vi "triangle.vi"() -> ()   [LabVIEW 2010]
panel:
  out "x galvo control true":u16(graph)
  out "x galvo control":u16(graph)
  in  "y resolution":u16
  out "control line counter":u16
  in  "stop":bool
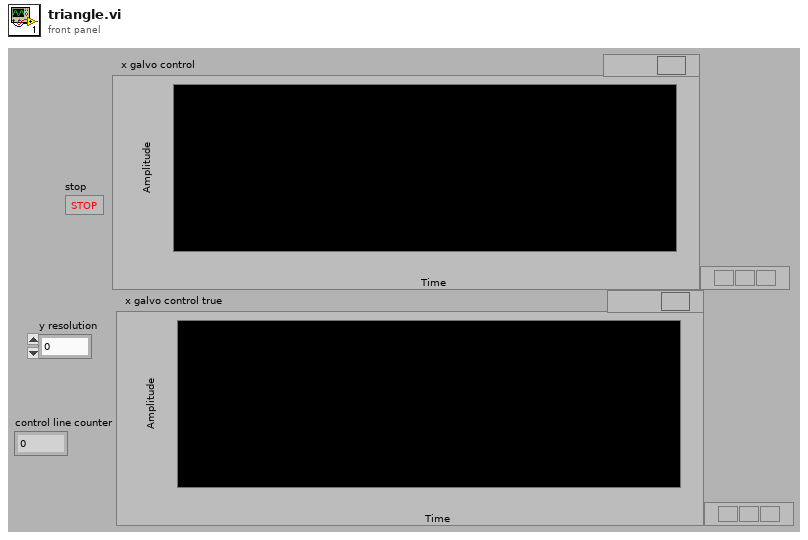
[diagram p1: front panel]
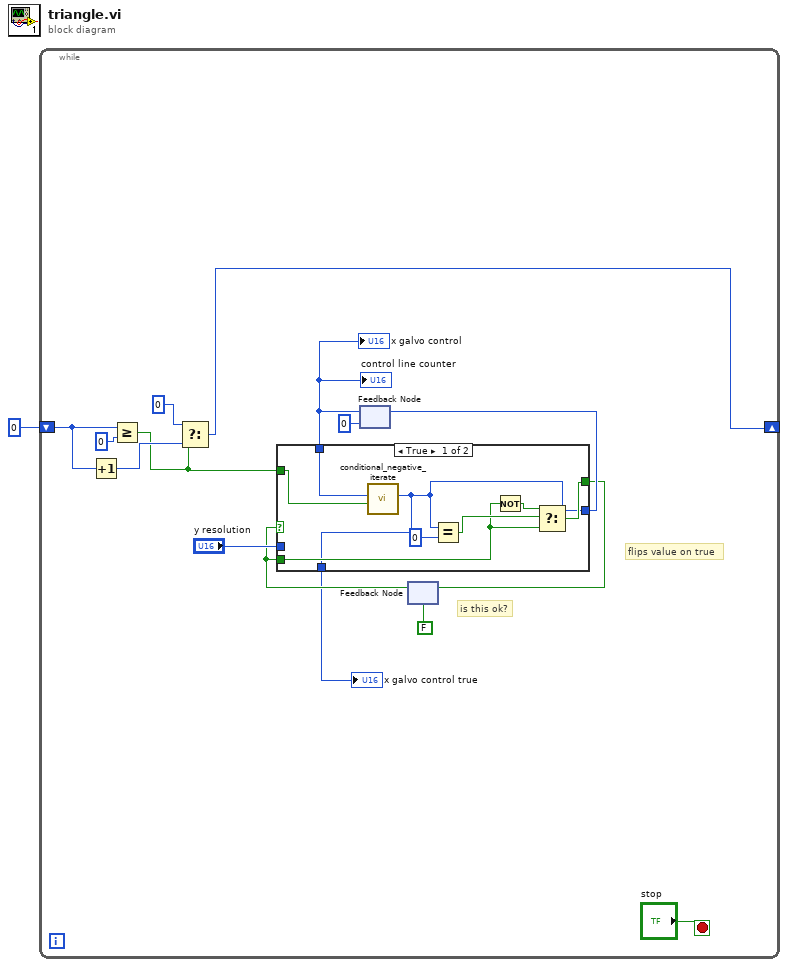
[diagram p0: block diagram]
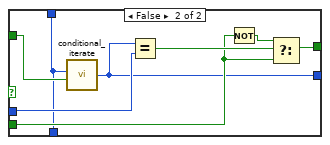
[diagram p2: hidden frame]
diagram:
  n1 = while {
    shift-right: [w12] -> _
    shift-left: u16 0 ("y") -> [w13]
    stop <- "stop" stop-if-true
    # "is this ok?"
    # "flips value on true"
    n2 = Increment(x=w13) -> (x+1=w5:u16)
    n3 = Greater Or Equal?(x=w13, y=u16 0) -> (x >= y?=w4:bool)
    n4 = Select(t=u16 0, s=w4, f=w5) -> (s? t:f=w12:u16)
    n5 = feedback #1(u16 0 ("number out")) -> (w10:u16)
    "control line counter" <- w10
    "x galvo control" <- w10
    n6 = feedback #2(FALSE) -> (w6:bool)
    n7 = case shown="True" w6 {
      tunnel: w4 -> [w23 w31]
      tunnel: "y resolution" -> [_ w27]
      tunnel: w10 -> [w18 w25]
      tunnel: [w17 w26] -> w9
      tunnel: [w21 w29] -> w7
      tunnel: w6 -> [w19 w28]
      tunnel: [w17 w25] -> w2
      frame True {
        n8 = call "conditional_negative_iterate.vi"("iterate?"=w23, "number in"=w18) -> ("number out"=w17:u16)  [unwired: 4 in]
        n9 = Equal?(x=w17, y=u16 0) -> (x = y?=w20:bool)
        n10 = Not(x=w19) -> (.not. x?=w22:bool)
        n11 = Select(t=w22, s=w20, f=w19) -> (s? t:f=w21:bool)
      }
      frame False {
        n12 = call "conditional_iterate.vi"("iterate?"=w31, "number in"=w25) -> ("number out"=w26:u16)  [unwired: 4 in]
        n13 = Equal?(x=w26, y=w27) -> (x = y?=w30:bool)
        n14 = Not(x=w28) -> (.not. x?=w32:bool)
        n15 = Select(t=w32, s=w30, f=w28) -> (s? t:f=w29:bool)
      }
    }
    "x galvo control true" <- w2
    n16 = feedback-in #1(w9) -> ()
    n17 = feedback-in #2(w7) -> ()
  }
